vi "Module-Delete.vi"(8 "error in":errorcluster, 11 "Name":string="4032248904914") -> (0 "error out":errorcluster)   [LabVIEW 2015, in "Settings-Style.lvlib"]
uses:
  Settings-Style.lvlib
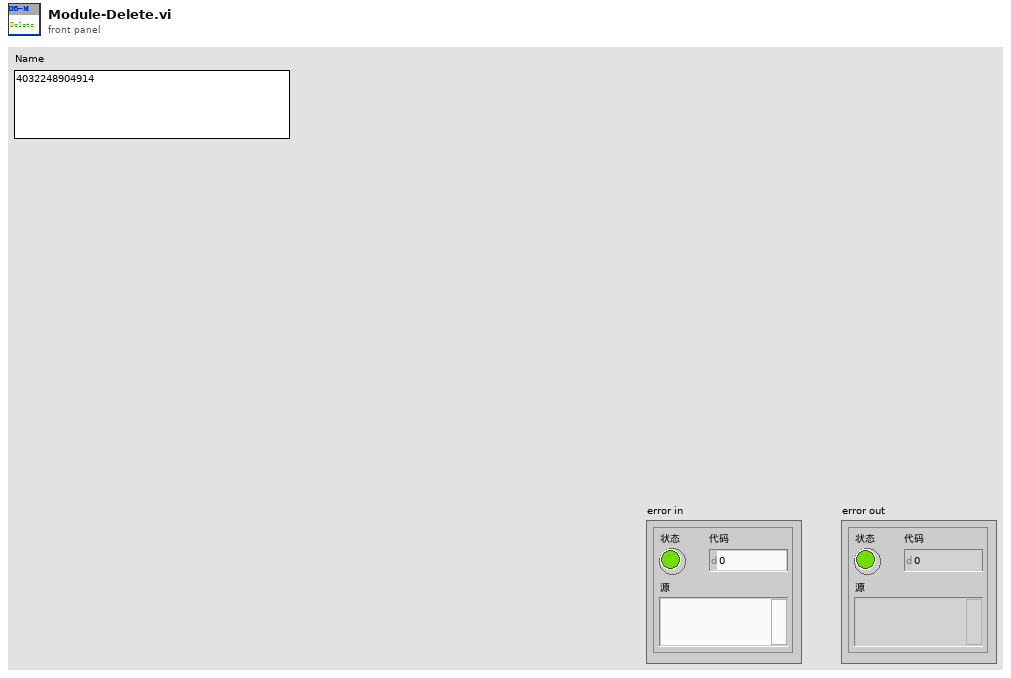
[diagram p1: front panel]
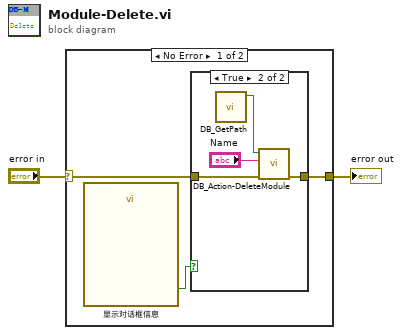
[diagram p0: block diagram]
diagram:
  n1 = case shown="No Error" "error in" {
    selector: "error in" -> [w4 w11]
    tunnel: [w3 w11] -> w2
    frame No Error {
      n2 = call "显示对话框信息"() -> ("确定 Done"=w5:bool)  [unwired: 10 in, 1 out]
      n3 = case shown="True" w5 {
        tunnel: w4 -> [w6 w10]
        tunnel: [w6 w9] -> w3
        frame False {
        }
        frame True {
          n4 = call "DB_GetPath.vi"() -> ("appended path"=w7:path)  [unwired: 11 in]
          n5 = call "DB_Action-DeleteModule.vi"("error in"=w10, "Name"="Name", "路径"=w7) -> ("error out"=w9:errorcluster)  [unwired: 8 in]
        }
      }
    }
    frame Error {
    }
  }
  "error out" <- w2
